vi "groundtest.vi"() -> ()   [LabVIEW 2011]
uses:
  <vilib>/Instr/_visa.llb/VISA Set IO Buffer Mask.ctl
  <vilib>/Instr/_visa.llb/VISA Configure Serial Port (Instr).vi
panel:
  in  "Logging ON":bool
  in  "Save to file":string
  out "Bad GPS Data":bool
  out "Bad Wind Data":bool
  out "Too much Roll":bool
  out "Bad Compass Data":bool
  out "Old Data":bool
  out "Checksum Bad":bool
  out "Two Commas":bool
  out "Rollover Data":bool
  out "No Data":bool
  out "ROLL":dbl(knob) scale=-45.0..45.0
  out "Time":string
  out "Right":bool
  out "Left":bool
  out "Tacking":bool
  out "Relative Wind Speed":dbl(knob) scale=0.0..15.0
  out "OUTPUT":string
  in  "Send":bool
  in  "INPUT":string
  out "Course/Bearing":cluster{i16, i16}(knob) scale=0.0..360.0 scale format="%.0f°"
  out "Distance":string
  out "RUDDER":dbl(knob) scale=-45.0..45.0
  out "MAIN":dbl(knob) scale=0.0..100.0
  out "GPS":bool
  in  "Baud Rate":string(combo)="9600"
  out "Batt":dbl format="%#_g V"
  out "LIPO":sgl(slide) scale=9.0..12.6 scale format="%#_g V"
  in  "quit?":bool
  in  "WaitForExit":bool
  in  "Launch EXE":bool
  out "Lat":dbl format="%.6g°"
  out "Lon":dbl format="%.6g°"
  in  "Choose Port":refnum<visa-resource-name>="COM5"
  out "True/ Rel":cluster{i16, i16}(knob) scale=0.0..360.0 scale format="%.0f°"
  out "Ground Speed":i32 format="%.0f m/s"
  out "error out":errorcluster={"status"=TRUE, "code"=-1073807346, "source"="VISA Read in groundtest.vi"}
  out "Part1":string
  # "QMAST"
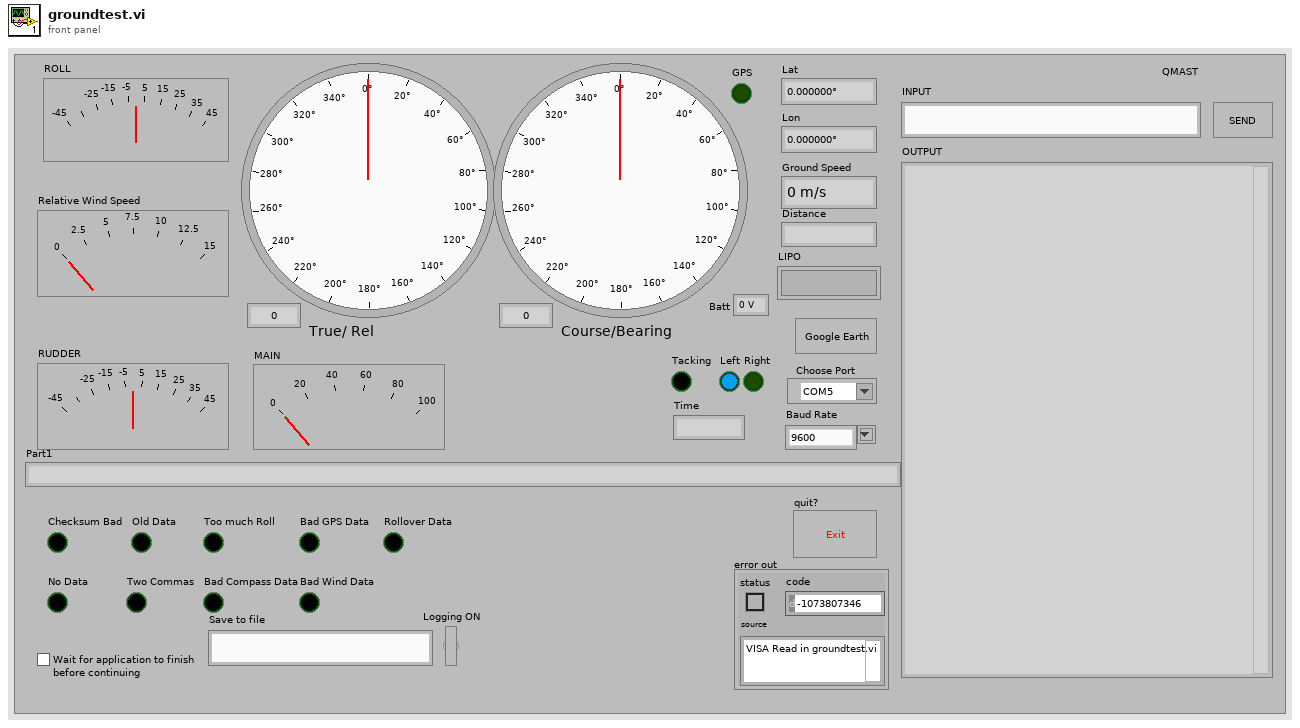
[diagram p1: front panel]
types:
  T1 = enum8{"Enabled", "Disabled", "Disabled and Grayed Out"}
  T2 = enum16{"open", "replace", "create", "open or create", "replace or create", "replace or create with confirmation"}
  T3 = typedef "VISA Set IO Buffer Mask.ctl" = u16
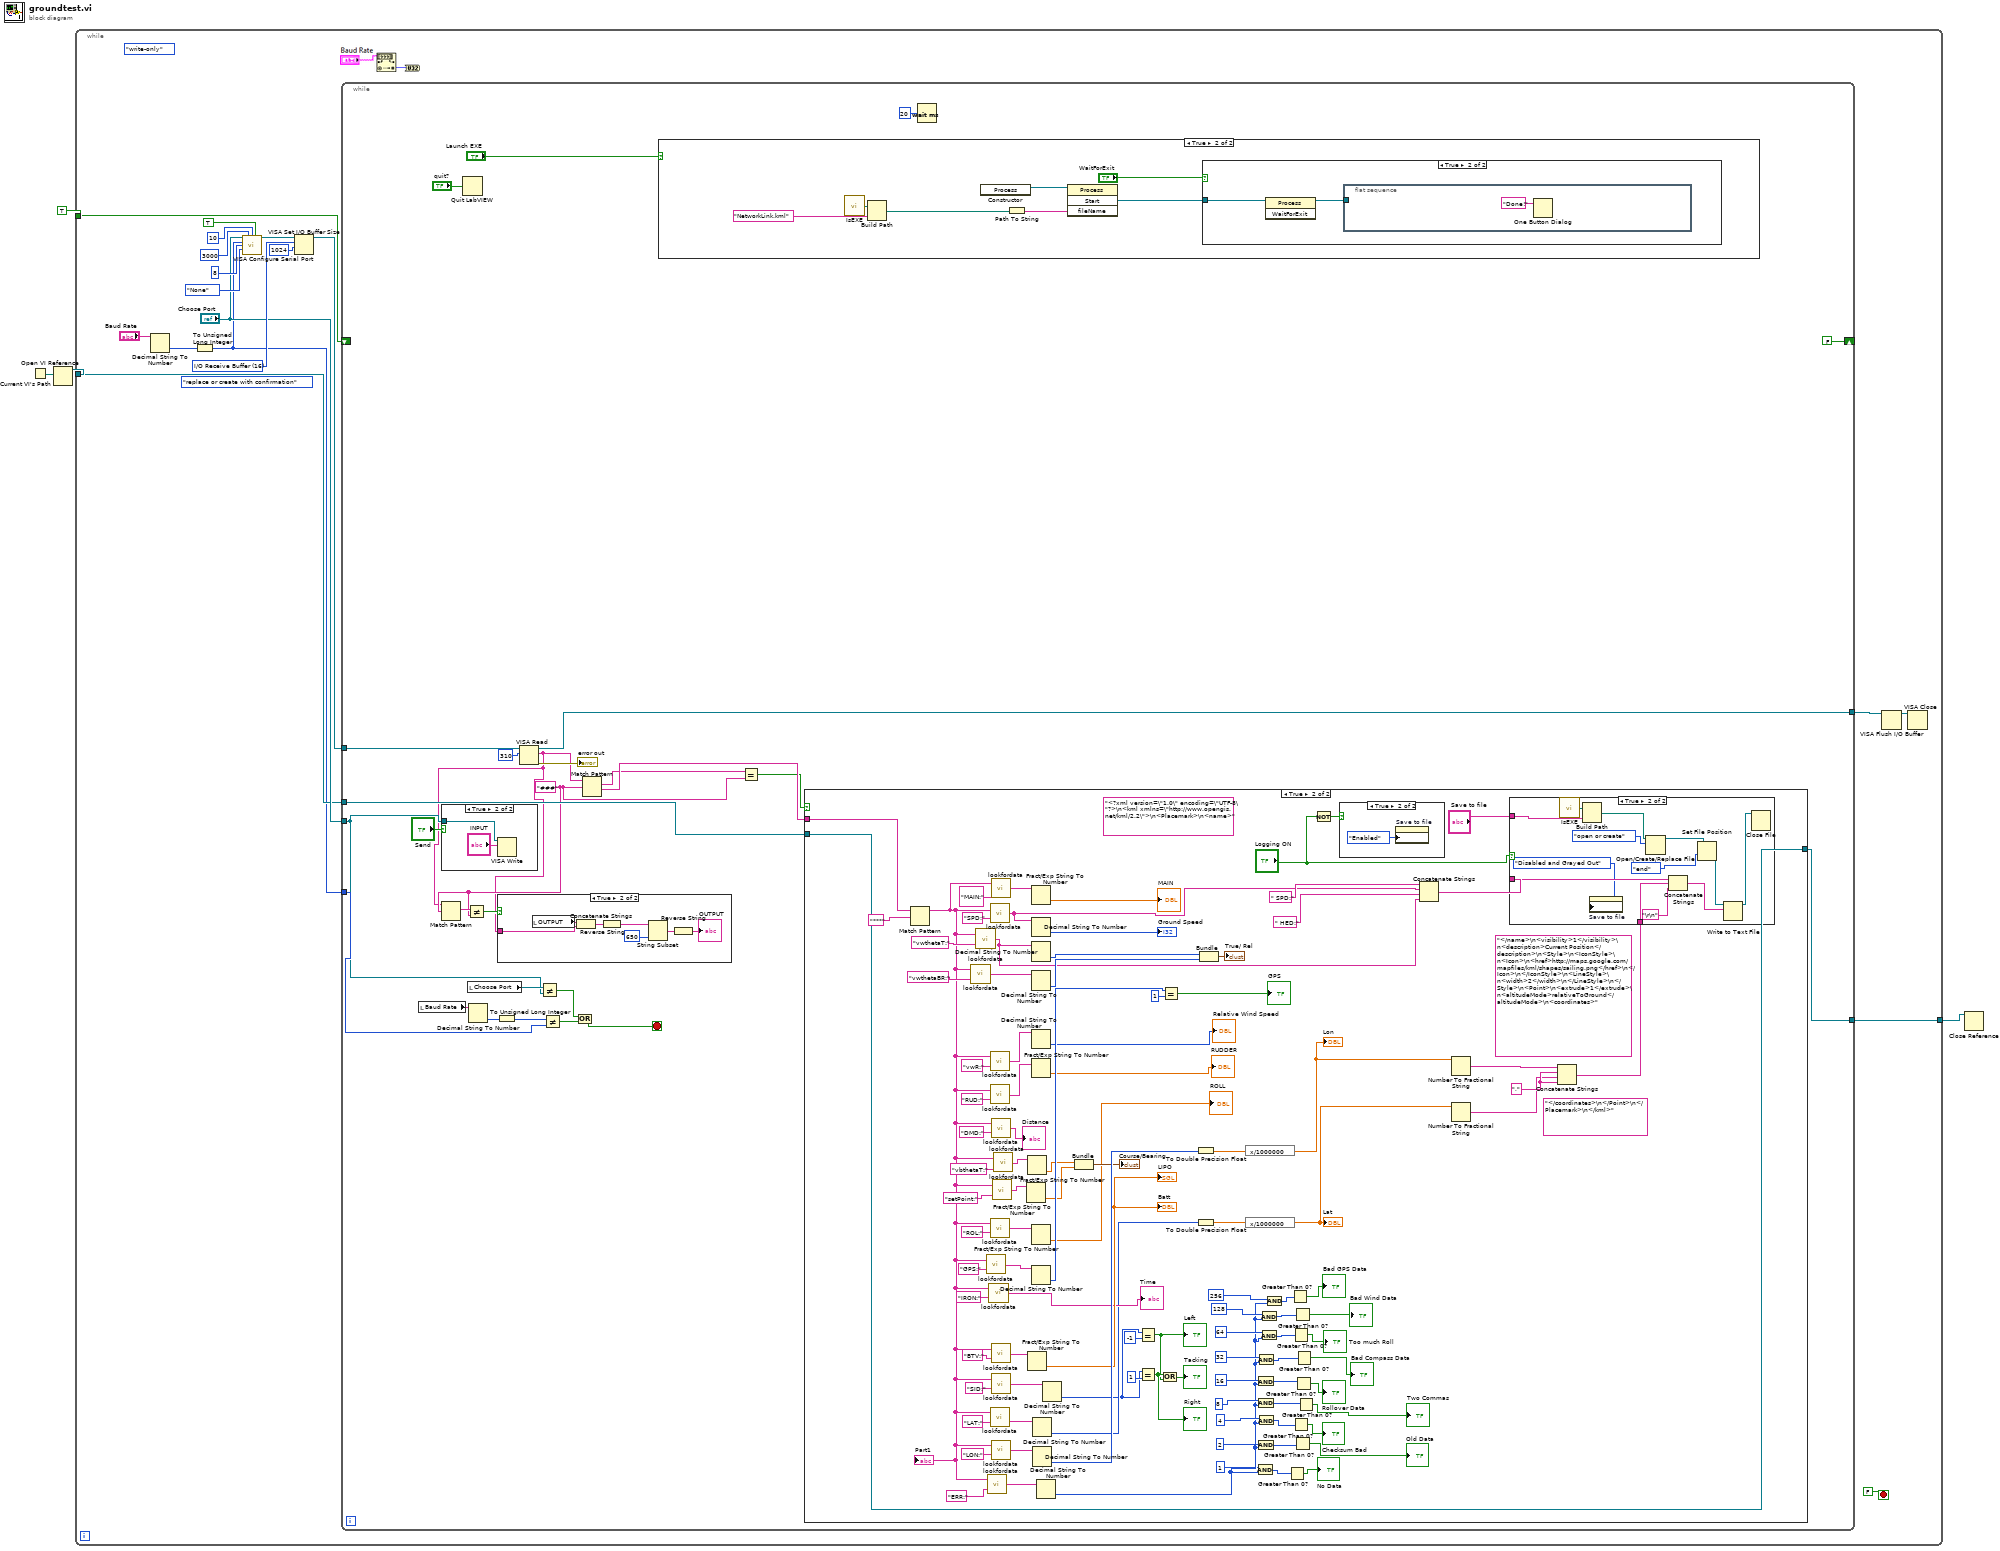
[diagram p0: block diagram]
diagram:
  n1 = Current VI's Path() -> (path=w2:path)
  n2 = Open VI Reference(vi path=w2) -> (vi reference=w1:refnum<vi>)  [unwired: 1 in, 5 out]
  n3 = while {
    tunnel: TRUE -> [w11]
    tunnel: [w10] -> w3
    tunnel: w1 -> [w9]
    stop <- FALSE stop-if-true
    (unwired) enum16{"read/write", "read-only", "write-only"}."write-only" ("access (0:read/write)")
    (unwired) T2."replace or create with confirmation" ("operation (0:open)")
    w23 = T3 16 items=["I/O Receive Buffer"=16, "I/O Transmit Buffer"=32, "I/O Receive and Transmit Buffer"=48] ("Mask")
    n4 = Decimal String To Number(string="Baud Rate") -> (number=w7:i32)  [unwired: 3 out]
    n5 = To Unsigned Long Integer(number=w7) -> (unsigned 32bit integer=w6:u32)
    n6 = call-poly "VISA Configure Serial Port"("VISA resource name"="Choose Port", "timeout (10sec)"=u32 3000, "termination char\n(0xA = '\\n' = LF)"=u8 10 ("termination char\n(0xA = '\\n' = LF)"), "Enable Termination\nChar (T)"=TRUE ("Enable Termination\nChar (T)"), "baud rate (9600)"=w6, "data bits (8)"=u16 8, "parity (0:none)"=enum16{"None", "Odd", "Even", "Mark", "Space"}."None") -> ("VISA resource name out"=w14:refnum<visa-resource-name>)  [unwired: 2 in, 6 out]
    n7 = VISA Set I/O Buffer Size(VISA resource name=w14, mask (16)=w23, size (4096)=u32 1024) -> (VISA resource name out=w5:refnum<visa-resource-name>)  [unwired: 1 in, 1 out]
    n8 = while {
      tunnel: w5 -> [w49]
      tunnel: [w48] -> w21
      tunnel: "Choose Port" -> [w29]
      shift-right: [FALSE] -> _
      shift-left: w11 -> [_]
      tunnel: [w38] -> w10
      tunnel: w9 -> [w37]
      tunnel: w6 -> [w36]
      stop <- w33 stop-if-true
      w26 = "###" ("regular expression")
      n9 = local read "Baud Rate"() -> (w31:string)
      n10 = case shown="True" "Send" {
        tunnel: w29 -> [_ w58]
        frame False {
        }
        frame True {
          n11 = VISA Write(VISA resource name=w58, write buffer="INPUT") -> ()  [unwired: 1 in, 3 out]
        }
      }
      n12 = Quit LabVIEW(quit? (T)="quit?") -> ()
      n13 = local read "Choose Port"() -> (w41:refnum<visa-resource-name>)
      n14 = Decimal String To Number(string=w31) -> (number=w32:i32)  [unwired: 3 out]
      n15 = To Unsigned Long Integer(number=w32) -> (unsigned 32bit integer=w30:u32)
      n16 = VISA Read(VISA resource name=w49, byte count=u32 310) -> (VISA resource name out=w48:refnum<visa-resource-name>, read buffer=w24:string, error out=→"error out":errorcluster)  [unwired: 1 in, 1 out]
      n17 = Match Pattern(string=w24, regular expression=w26) -> (match substring=w27:string)  [unwired: 1 in, 3 out]
      n18 = Not Equal?(x=w27, y=w26) -> (x != y?=w25:bool)
      n19 = case shown="True" w25 {
        tunnel: w24 -> [_ w55]
        frame False {
        }
        frame True {
          n20 = local read "OUTPUT"() -> (w56:string)
          n21 = Concatenate Strings(w56, w55) -> (w54:string)
          n22 = Reverse String(1:w54) -> (0:w53:string)
          n23 = String Subset(string=w53, length (rest)=650) -> (substring=w52:string)  [unwired: 1 in]
          n24 = Reverse String(1:w52) -> (0:→"OUTPUT":string)
        }
      }
      n25 = Not Equal?(x=w41, y=w29) -> (x != y?=w35:bool)
      n26 = Not Equal?(x=w30, y=w36) -> (x != y?=w34:bool)
      n27 = Or(x=w35, y=w34) -> (x .or. y?=w33:bool)
      n28 = Match Pattern(string=w24, regular expression=w26) -> (match substring=w43:string, after substring=w50:string)  [unwired: 3 out]
      n29 = case shown="True" "Launch EXE" {
        frame False {
        }
        frame True {
          n30 = call "IsEXE.vi"() -> ("path to vi or exe install\\data\\ dir"=w60:path)  [unwired: 10 out]
          n31 = Build Path(base path=w60, name or relative path="NetworkLink.kml") -> (appended path=w61:path)
          n32 = constructor class="Process"() -> (reference out=w66:refnum<k24>)  [unwired: 3 in, 2 out]
          n33 = Path To String(path=w61) -> (string=w65:string)
          n34 = invoke class="Process" method="Start"(reference=w66, "fileName"=w65) -> ("Start"=w64:refnum<k24>)  [unwired: 2 in, 3 out]
          n35 = case shown="True" "WaitForExit" {
            tunnel: w64 -> [_ w68]
            frame False {
            }
            frame True {
              n36 = invoke class="Process" method="WaitForExit"(reference=w68) -> (reference out=w67:refnum<k24>)  [unwired: 2 in, 2 out]
              n37 = flat-sequence {
                tunnel: w67 -> [_]
                frame #0 {
                  n38 = One Button Dialog(message="Done!") -> ()  [unwired: 2 out]
                }
              }
            }
          }
        }
      }
      n39 = Equal?(x=w43, y=w26) -> (x = y?=w44:bool)
      n40 = case shown="True" w44 {
        tunnel: w50 -> [_ w149]
        tunnel: [_ w112] -> w38
        tunnel: w37 -> [_ w112]
        frame False {
        }
        frame True {
          (unwired) "</name>\n<visibility>1</visibility>\n<description>Current Position</description>\n<Style>\n<IconStyle>\n<Icon>\n<href>http://maps.google.com/mapfiles/kml/shapes/sailing.png</href>\n</Icon>\n</IconStyle>\n<LineStyle>\n<width>2</width>\n</LineStyle>\n</Style>\n<Point>\n<extrude>1</extrude>\n<altitudeMode>relativeToGround</altitudeMode>\n<coordinates>"
          w158 = ","
          (unwired) "</coordinates>\n</Point>\n</Placemark>\n</kml>"
          (unwired) "<?xml version=\"1.0\" encoding=\"UTF-8\"?>\n<kml xmlns=\"http://www.opengis.net/kml/2.2\">\n<Placemark>\n<name>"
          n41 = Match Pattern(string=w149, regular expression="***") -> (before substring=w70:string)  [unwired: 4 out]
          "Part1" <- w70
          n42 = call "lookfordata.vi"("Header"="vwthetaBR:", "string"=w70) -> ("output string"=w140:string)
          n43 = call "lookfordata.vi"("Header"="vwthetaT:", "string"=w70) -> ("output string"=w71:string)
          n44 = call "lookfordata.vi"("Header"="GPS:" ("regular expression"), "string"=w70) -> ("output string"=w170:string)
          n45 = call "lookfordata.vi"("Header"="ERR:", "string"=w70) -> ("output string"=w109:string)
          n46 = call "lookfordata.vi"("Header"="IRON:", "string"=w70) -> ("output string"=→"Time":string)
          n47 = call "lookfordata.vi"("Header"="SPD:", "string"=w70) -> ("output string"=w73:string)
          n48 = call "lookfordata.vi"("Header"="vwR:", "string"=w70) -> ("output string"=w129:string)
          n49 = call "lookfordata.vi"("Header"="RUD:", "string"=w70) -> ("output string"=w134:string)
          n50 = call "lookfordata.vi"("Header"="ROL:", "string"=w70) -> ("output string"=w142:string)
          n51 = call "lookfordata.vi"("Header"="LAT:", "string"=w70) -> ("output string"=w159:string)
          n52 = call "lookfordata.vi"("Header"="MAIN:", "string"=w70) -> ("output string"=w135:string)
          n53 = call "lookfordata.vi"("Header"="DMD:", "string"=w70) -> ("output string"=→"Distance":string)
          n54 = call "lookfordata.vi"("Header"="BTV:", "string"=w70) -> ("output string"=w147:string)
          n55 = call "lookfordata.vi"("Header"="SID:", "string"=w70) -> ("output string"=w118:string)
          n56 = call "lookfordata.vi"("Header"="LON:", "string"=w70) -> ("output string"=w161:string)
          n57 = call "lookfordata.vi"("Header"="setPoint:", "string"=w70) -> ("output string"=w124:string)
          n58 = call "lookfordata.vi"("Header"="vbthetaT:", "string"=w70) -> ("output string"=w125:string)
          n59 = Fract/Exp String To Number(string=w124) -> (number=w123:dbl)  [unwired: 4 out]
          n60 = Fract/Exp String To Number(string=w147) -> (number=→"LIPO" →"Batt":dbl)  [unwired: 4 out]
          n61 = Fract/Exp String To Number(string=w125) -> (number=w122:dbl)  [unwired: 4 out]
          n62 = Fract/Exp String To Number(string=w135) -> (number=→"MAIN":dbl)  [unwired: 4 out]
          n63 = Decimal String To Number(string=w73) -> (number=→"Ground Speed":i32)  [unwired: 3 out]
          n64 = Decimal String To Number(string=w71) -> (number=w169:i32)  [unwired: 3 out]
          n65 = Decimal String To Number(string=w140) -> (number=w168:i32)  [unwired: 3 out]
          n66 = Decimal String To Number(string=w129) -> (number=→"Relative Wind Speed":i32)  [unwired: 3 out]
          n67 = Fract/Exp String To Number(string=w134) -> (number=→"RUDDER":dbl)  [unwired: 4 out]
          n68 = Fract/Exp String To Number(string=w142) -> (number=→"ROLL":dbl)  [unwired: 4 out]
          n69 = Decimal String To Number(string=w170) -> (number=w144:i32)  [unwired: 3 out]
          n70 = Decimal String To Number(string=w159) -> (number=w115:i32)  [unwired: 3 out]
          n71 = Decimal String To Number(string=w161) -> (number=w152:i32)  [unwired: 3 out]
          n72 = Decimal String To Number(string=w109) -> (number=w85:i32)  [unwired: 3 out]
          n73 = Decimal String To Number(string=w118) -> (number=w113:i32)  [unwired: 2 in, 1 out]
          n74 = Bundle(w122, w123) -> (→"Course/Bearing":cluster{dbl, dbl})  [unwired: 1 out]
          n75 = Equal?(x=w113, y=-1) -> (x = y?=w78:bool)
          "Left" <- w78
          n76 = Equal?(x=w113, y=1) -> (x = y?=w79:bool)
          "Right" <- w79
          n77 = Or(x=w79, y=w78) -> (x .or. y?=→"Tacking":bool)
          n78 = Equal?(x=w144, y=1) -> (x = y?=→"GPS":bool)
          n79 = To Double Precision Float(number=w152) -> (double precision float=w154:dbl)
          n80 = To Double Precision Float(number=w115) -> (double precision float=w153:dbl)
          n81 = Bundle(w169, w168) -> (→"True/ Rel":cluster{i32, i32})  [unwired: 1 out]
          n82 = expression code="x/1000000"(w154) -> (w151:dbl)
          "Lon" <- w151
          n83 = expression code="x/1000000"(w153) -> (w150:dbl)
          "Lat" <- w150
          n84 = And(x=1, y=w85) -> (x .and. y?=w101:i32)
          n85 = And(x=16, y=w85) -> (x .and. y?=w96:i32)
          n86 = And(x=8, y=w85) -> (x .and. y?=w95:i32)
          n87 = And(x=2, y=w85) -> (x .and. y?=w81:i32)
          n88 = And(x=32, y=w85) -> (x .and. y?=w97:i32)
          n89 = And(x=4, y=w85) -> (x .and. y?=w94:i32)
          n90 = And(x=128, y=w85) -> (x .and. y?=w99:i32)
          n91 = And(x=64, y=w85) -> (x .and. y?=w98:i32)
          n92 = And(x=256, y=w85) -> (x .and. y?=w84:i32)
          n93 = Greater Than 0?(x=w101) -> (x > 0?=→"No Data":bool)
          n94 = Greater Than 0?(x=w84) -> (x > 0?=→"Bad GPS Data":bool)
          n95 = Greater Than 0?(x=w98) -> (x > 0?=→"Too much Roll":bool)
          n96 = Greater Than 0?(x=w94) -> (x > 0?=→"Checksum Bad":bool)
          n97 = Greater Than 0?(x=w99) -> (x > 0?=→"Bad Wind Data":bool)
          n98 = Greater Than 0?(x=w81) -> (x > 0?=→"Old Data":bool)
          n99 = Greater Than 0?(x=w96) -> (x > 0?=→"Rollover Data":bool)
          n100 = Greater Than 0?(x=w97) -> (x > 0?=→"Bad Compass Data":bool)
          n101 = Greater Than 0?(x=w95) -> (x > 0?=→"Two Commas":bool)
          n102 = Not(x="Logging ON") -> (.not. x?=w74:bool)
          n103 = case shown="True" w74 {
            frame False {
            }
            frame True {
              n104 = property on="Save to file" class="Str"("DisabledEnum"=T1."Enabled" ("Disabled")) -> ()  [unwired: 2 in, 2 out]
            }
          }
          n105 = Concatenate Strings "Concatenate Strings"(" SPD:", w73, " HED:", w71) -> (w77:string)
          n106 = Number To Fractional String(number=w151) -> (F-format string=w157:string)  [unwired: 3 out]
          n107 = Number To Fractional String(number=w150) -> (F-format string=w156:string)  [unwired: 3 out]
          n108 = Concatenate Strings(w157, w158, w156, w158) -> (w155:string)
          n109 = case shown="True" "Logging ON" {
            tunnel: w155 -> [_ w182]
            tunnel: w77 -> [_ w180]
            tunnel: "Save to file" -> [_ w175]
            frame False {
            }
            frame True {
              n110 = call "IsEXE.vi"() -> ("path to vi or exe install\\data\\ dir"=w181:path)  [unwired: 10 out]
              n111 = Build Path(base path=w181, name or relative path=w175) -> (appended path=w186:path)
              n112 = property on="Save to file" class="Str"("DisabledEnum"=T1."Disabled and Grayed Out" ("Disabled")) -> ()  [unwired: 2 in, 2 out]
              n113 = Open/Create/Replace File(file path (use dialog)=w186, operation (0:open)=T2."open or create") -> (refnum out=w178:refnum<file>)  [unwired: 2 in, 4 out]
              n114 = Concatenate Strings(w180, w182, "\r\n") -> (w184:string)
              n115 = Set File Position(refnum=w178, from (0:start)=enum16{"start", "end", "current"}."end") -> (refnum out=w177:refnum<file>)  [unwired: 2 in, 1 out]
              n116 = Write to Text File(file (use dialog)=w177, text=w184) -> (refnum out=w183:refnum<file>)  [unwired: 1 in, 3 out]
              n117 = Close File(refnum=w183) -> ()  [unwired: 1 in, 2 out]
            }
          }
        }
      }
      n118 = Wait (ms)(milliseconds to wait=u32 20) -> ()  [unwired: 1 out]
    }
    n119 = VISA Flush I/O Buffer(VISA resource name=w21) -> (VISA resource name out=w20:refnum<visa-resource-name>)  [unwired: 1 in, 2 out]
    n120 = VISA Close(VISA resource name=w20) -> ()  [unwired: 1 in, 1 out]
  }
  n121 = Close Reference(reference=w3) -> ()  [unwired: 1 in, 1 out]
